vi "Look for table in database.vi"(8 "error in (no error)":errorcluster, 10 "Table Name":string, 11 "connection reference":T1) -> (0 "error out":errorcluster, 1 "tables in database":string[](array[string]), 2 "table found in database":bool, 3 "connection reference out":T1)   [LabVIEW 2023, in "SQL Database.lvlib"]
uses:
  <vilib>/addons/database/Connection.llb/Conn ObjectReference.ctl
  SQL Database.lvlib
  <vilib>/addons/database/NI_Database_API.lvlib
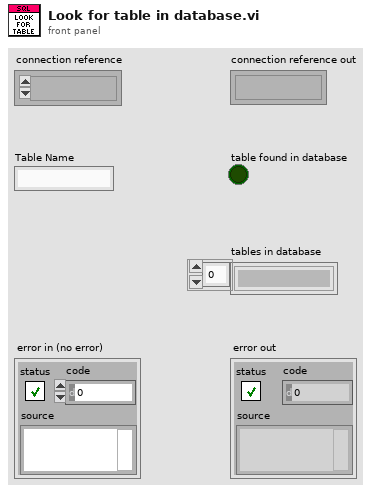
[diagram p1: front panel]
types:
  T1 = typedef "NI_Database_API.lvlib/Conn ObjectReference.ctl" = refnum<k1>
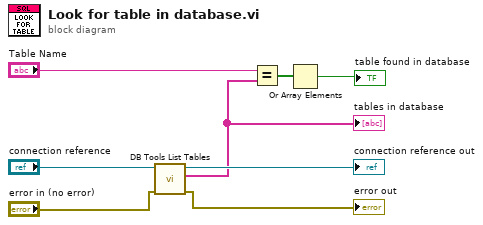
[diagram p0: block diagram]
diagram:
  n1 = call <vilib>:"DB Tools List Tables.vi"("error in (no error)"="error in (no error)", "connection reference"="connection reference") -> ("error out"=→"error out":errorcluster, "tables"=w6:string[], "connection reference out"=→"connection reference out":T1)  [unwired: 3 in]
  "tables in database" <- w6
  n2 = Equal?(x="Table Name", y=w6) -> (x = y?=w4:bool[])
  n3 = Or Array Elements(Boolean array=w4) -> (logical OR=→"table found in database":bool)
